vi "RSNRPZ Get Correction Frequency Step.vi"(8 "error in (no error)":errorcluster, 9 "Channel (1)":i32=1, 11 "VISA session":refnum<visa-resource-name> caption="VISA resource name") -> (0 "error out":errorcluster, 2 "Frequency Step":dbl format="%^.3e", 3 "dup VISA session":refnum<visa-resource-name> caption="VISA resource name")   [LabVIEW 2010]
doc: "This VI returns the frequency step value.\n\nRemote-control command(s):\nSENS:FREQ:STEP?"
uses:
  rsnrpz_32.dll
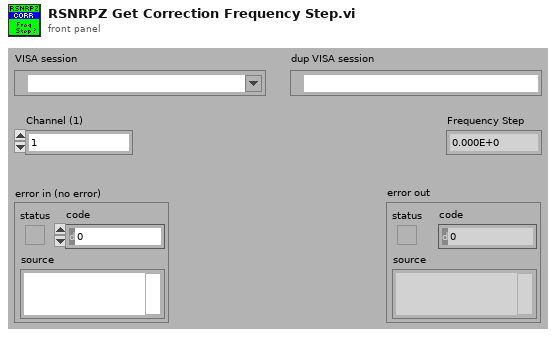
[diagram p1: front panel]
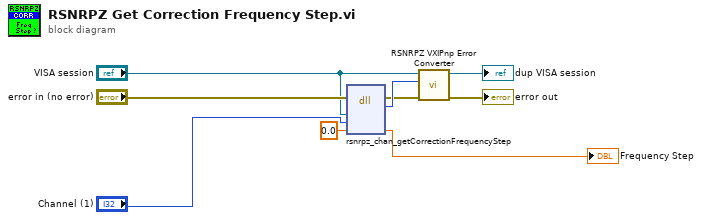
[diagram p0: block diagram]
diagram:
  n1 = dll-call lib="rsnrpz_32.dll" fn="rsnrpz_chan_getCorrectionFrequencyStep"(error in="error in (no error)", "Instrument Handle"="VISA session", "Channel"="Channel (1)", "Frequency Step"=0.0) -> (error out=w5:errorcluster, w7:i32, "Frequency Step"=→"Frequency Step":dbl)  [unwired: 4 in, 1 out]
  n2 = call <instrlib>:"RSNRPZ VXIPnp Error Converter.vi"("error in"=w5, "VXIPnp error code"=w7, "VISA session"="VISA session") -> ("error out"=→"error out":errorcluster, "dup VISA session"=→"dup VISA session":refnum<visa-resource-name>)  [unwired: 7 in]
